vi "test_libssh2_session_callback_set.vi"() -> ()   [LabVIEW 2017, in "integration_tests.lvlib"]
uses:
  integration_tests.lvlib
  libssh2/libssh2_session_abstract.ctl
  libssh2/libssh2_session_callback_type.ctl
  libssh2/libssh2_session_handshake_tcp.vi
  libssh2/libssh2_init_default.vi
  <vilib>/Utility/tcp.llb/TCP Get Raw Net Object.vi
  libssh2/libssh2_session_handshake_socket.vi
  libssh2/libssh2_session_disconnect_ex.vi
  libssh2/libssh2.lvlib
  support/support.lvlib
  <vilib>/PNR/Transparent Assertions/Transparent Assertions/Transparent Assertions.lvlib
panel:
  out "error out":errorcluster
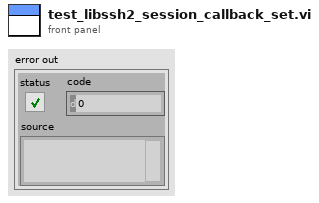
[diagram p1: front panel]
types:
  T1 = typedef "libssh2.lvlib/libssh2_session_abstract.ctl" = cluster{"send":refnum<vi>, "receive":refnum<vi>, "keyboard-interactive response":refnum<vi>}
  T2 = typedef "libssh2.lvlib/Session Refnum.ctl" = refnum<k1>
  T3 = typedef "libssh2.lvlib/libssh2_session_callback_type.ctl" = enum16{"Ignore", "Debug", "Disconnect", "MAC Error", "X11", "Send", "Receive", "Auth Agent", "Auth Agent Identities", "Auth Agent Sign"}
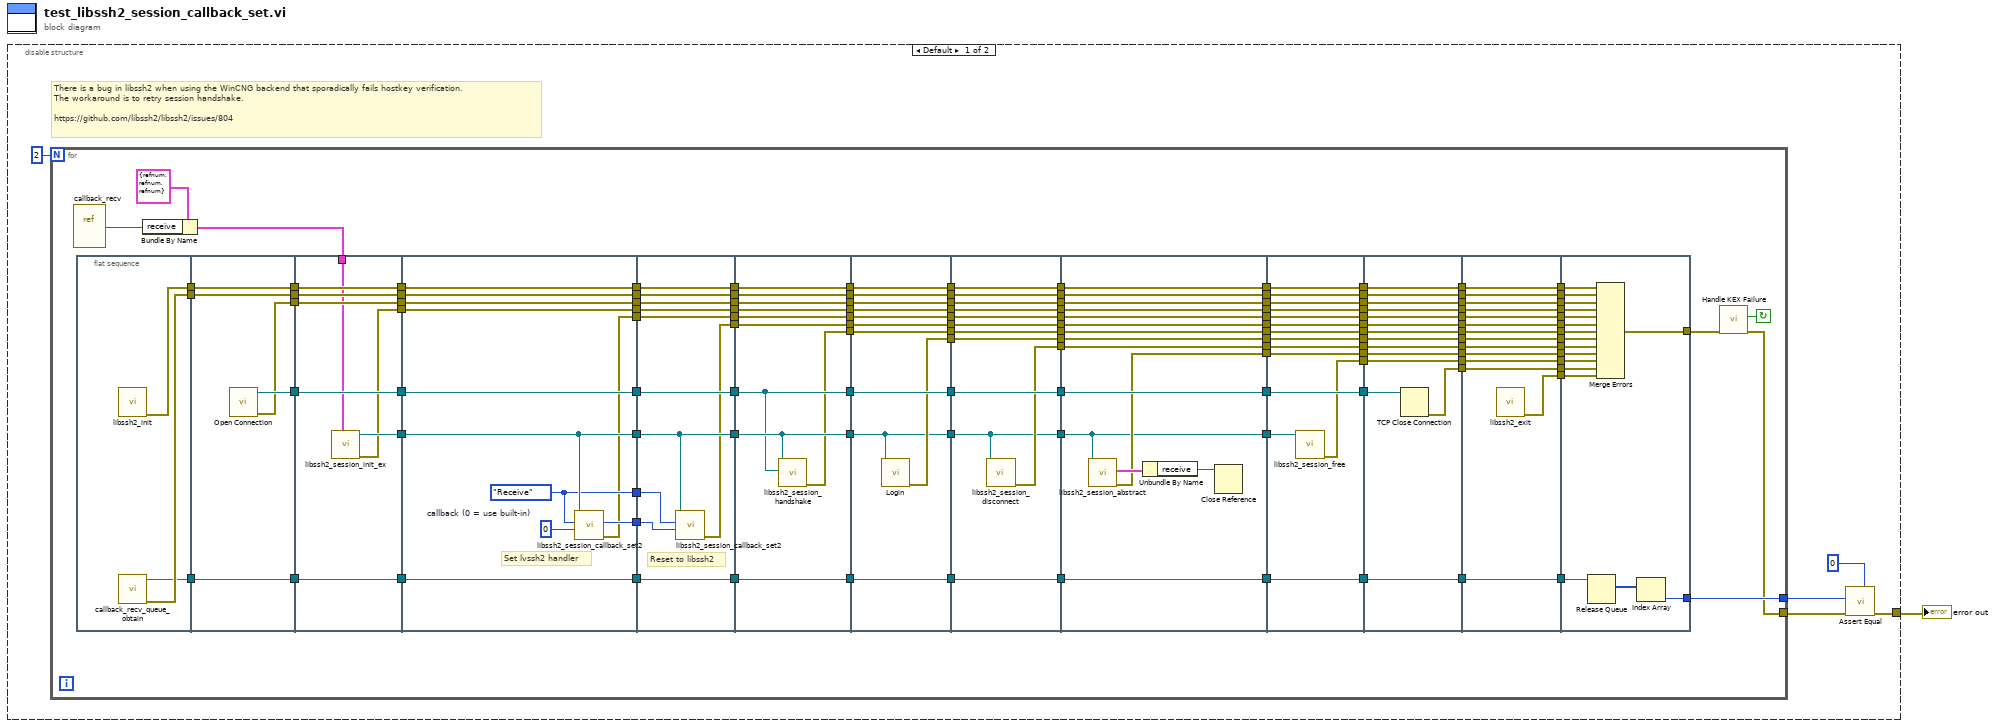
[diagram p0: block diagram]
diagram:
  n1 = disable-structure shown="Default" {
    disable-tunnel: [w5 _] -> w1
    frame condition #0 (active) {
      # "There is a bug in libssh2 when using the WinCNG backend that sporadically fails hostkey verification.\nThe workaround is to retry session handshake.\n\nhttps://github.com/libssh2/libssh2/issues/804"
      n2 = for {
        N: 2 -> [_]
        tunnel: [w10] -> w4
        tunnel: [w8] -> w3
        stop <- w7 continue-if-true
        n3 = vi-ref "callback_recv.vi"() -> (w12:refnum<vi>)
        n4 = flat-sequence {
          tunnel: [w136] -> w133
          tunnel: [w135] -> w132
          tunnel: [w134] -> w131
          tunnel: [w141] -> w130
          tunnel: w133 -> [w140]
          tunnel: [w140] -> w129
          tunnel: [w139] -> w128
          tunnel: w132 -> [w138]
          tunnel: [w138] -> w127
          tunnel: [w137] -> w126
          tunnel: w131 -> [w137]
          tunnel: w130 -> [w149]
          tunnel: [w149] -> w125
          tunnel: w129 -> [w148]
          tunnel: [w148] -> w124
          tunnel: w128 -> [w147]
          tunnel: [w147] -> w123
          tunnel: [w146] -> w122
          tunnel: [w145] -> w121
          tunnel: w127 -> [w144]
          tunnel: [w144] -> w120
          tunnel: w11 -> [w143]
          tunnel: [w142] -> w119
          tunnel: w126 -> [w142]
          tunnel: w125 -> [w160]
          tunnel: [w160] -> w118
          tunnel: w124 -> [w159]
          tunnel: [w159] -> w117
          tunnel: w123 -> [w158]
          tunnel: [w158] -> w116
          tunnel: w122 -> [w155]
          tunnel: [w155] -> w115
          tunnel: w121 -> [w157]
          tunnel: [w157] -> w114
          tunnel: w120 -> [w156]
          tunnel: [w156] -> w113
          tunnel: w119 -> [w154]
          tunnel: [w154] -> w112
          tunnel: [w153] -> w111
          tunnel: [w152] -> w110
          tunnel: [w151] -> w109
          tunnel: w118 -> [w171]
          tunnel: [w171] -> w108
          tunnel: w117 -> [w170]
          tunnel: [w170] -> w107
          tunnel: w116 -> [w169]
          tunnel: [w169] -> w106
          tunnel: w115 -> [w163]
          tunnel: [w163] -> w105
          tunnel: w114 -> [w168]
          tunnel: [w168] -> w104
          tunnel: w113 -> [w167]
          tunnel: [w167] -> w103
          tunnel: w112 -> [w166]
          tunnel: [w166] -> w102
          tunnel: w111 -> [w165]
          tunnel: w110 -> [w164]
          tunnel: w109 -> [w162]
          tunnel: [w162] -> w101
          tunnel: [w161] -> w100
          tunnel: w108 -> [w177]
          tunnel: [w177] -> w99
          tunnel: w107 -> [w181]
          tunnel: [w181] -> w98
          tunnel: w106 -> [w180]
          tunnel: [w180] -> w97
          tunnel: [w179] -> w96
          tunnel: w105 -> [w179]
          tunnel: w104 -> [w178]
          tunnel: [w178] -> w95
          tunnel: [w176] -> w94
          tunnel: w103 -> [w175]
          tunnel: [w175] -> w93
          tunnel: [w174] -> w92
          tunnel: w102 -> [w174]
          tunnel: w101 -> [w173]
          tunnel: [w173] -> w91
          tunnel: w100 -> [w172]
          tunnel: [w172] -> w90
          tunnel: w99 -> [w192]
          tunnel: [w192] -> w89
          tunnel: w98 -> [w191]
          tunnel: [w191] -> w88
          tunnel: w97 -> [w190]
          tunnel: [w190] -> w87
          tunnel: w96 -> [w185]
          tunnel: w95 -> [w189]
          tunnel: [w189] -> w86
          tunnel: w94 -> [w188]
          tunnel: [w188] -> w85
          tunnel: w93 -> [w187]
          tunnel: [w187] -> w84
          tunnel: [w186] -> w83
          tunnel: [w185] -> w82
          tunnel: [w184] -> w81
          tunnel: w92 -> [w184]
          tunnel: w91 -> [w183]
          tunnel: [w183] -> w80
          tunnel: w90 -> [w182]
          tunnel: [w182] -> w79
          tunnel: w89 -> [w204]
          tunnel: [w204] -> w78
          tunnel: w88 -> [w203]
          tunnel: [w203] -> w77
          tunnel: w87 -> [w202]
          tunnel: [w202] -> w76
          tunnel: w86 -> [w201]
          tunnel: [w201] -> w75
          tunnel: [w200] -> w74
          tunnel: w85 -> [w199]
          tunnel: [w199] -> w73
          tunnel: w84 -> [w198]
          tunnel: [w198] -> w72
          tunnel: w83 -> [w197]
          tunnel: [w197] -> w71
          tunnel: [w196] -> w70
          tunnel: w82 -> [w196]
          tunnel: [w195] -> w69
          tunnel: w81 -> [w195]
          tunnel: w80 -> [w194]
          tunnel: [w194] -> w68
          tunnel: w79 -> [w193]
          tunnel: [w193] -> w67
          tunnel: w78 -> [w219]
          tunnel: [w219] -> w66
          tunnel: w77 -> [w218]
          tunnel: [w218] -> w65
          tunnel: w76 -> [w217]
          tunnel: [w217] -> w64
          tunnel: w75 -> [w216]
          tunnel: [w216] -> w63
          tunnel: w74 -> [w215]
          tunnel: [w215] -> w62
          tunnel: w73 -> [w214]
          tunnel: [w214] -> w61
          tunnel: w72 -> [w213]
          tunnel: [w213] -> w60
          tunnel: w71 -> [w212]
          tunnel: [w212] -> w59
          tunnel: w70 -> [w208]
          tunnel: [w209] -> w58
          tunnel: [w208] -> w57
          tunnel: [w207] -> w56
          tunnel: w69 -> [w207]
          tunnel: w68 -> [w206]
          tunnel: [w206] -> w55
          tunnel: w67 -> [w205]
          tunnel: [w205] -> w54
          tunnel: w66 -> [w233]
          tunnel: [w233] -> w53
          tunnel: w65 -> [w232]
          tunnel: [w232] -> w52
          tunnel: w64 -> [w231]
          tunnel: [w231] -> w51
          tunnel: w63 -> [w230]
          tunnel: [w230] -> w50
          tunnel: w62 -> [w229]
          tunnel: [w229] -> w49
          tunnel: w61 -> [w228]
          tunnel: [w228] -> w48
          tunnel: w60 -> [w227]
          tunnel: [w227] -> w47
          tunnel: w59 -> [w226]
          tunnel: [w226] -> w46
          tunnel: w58 -> [w225]
          tunnel: [w225] -> w45
          tunnel: w57 -> [w224]
          tunnel: [w223] -> w44
          tunnel: [w222] -> w43
          tunnel: w56 -> [w222]
          tunnel: w55 -> [w221]
          tunnel: [w221] -> w42
          tunnel: w54 -> [w220]
          tunnel: [w220] -> w41
          tunnel: w53 -> [w247]
          tunnel: w52 -> [w246]
          tunnel: [w246] -> w40
          tunnel: w51 -> [w245]
          tunnel: [w245] -> w39
          tunnel: [w244] -> w38
          tunnel: w50 -> [w243]
          tunnel: [w243] -> w37
          tunnel: w49 -> [w242]
          tunnel: [w242] -> w36
          tunnel: w48 -> [w241]
          tunnel: [w241] -> w35
          tunnel: w47 -> [w240]
          tunnel: [w240] -> w34
          tunnel: w46 -> [w239]
          tunnel: [w239] -> w33
          tunnel: w45 -> [w238]
          tunnel: [w238] -> w32
          tunnel: [w237] -> w31
          tunnel: w44 -> [w237]
          tunnel: [w236] -> w30
          tunnel: w43 -> [w236]
          tunnel: w42 -> [w235]
          tunnel: [w235] -> w29
          tunnel: w41 -> [w234]
          tunnel: [w234] -> w28
          tunnel: w40 -> [w261]
          tunnel: [w261] -> w27
          tunnel: w39 -> [w260]
          tunnel: [w260] -> w26
          tunnel: w38 -> [w259]
          tunnel: [w259] -> w25
          tunnel: [w258] -> w24
          tunnel: w37 -> [w257]
          tunnel: [w257] -> w23
          tunnel: w36 -> [w256]
          tunnel: [w256] -> w22
          tunnel: w35 -> [w255]
          tunnel: [w255] -> w21
          tunnel: w34 -> [w254]
          tunnel: [w254] -> w20
          tunnel: w33 -> [w253]
          tunnel: [w253] -> w19
          tunnel: w32 -> [w252]
          tunnel: [w252] -> w18
          tunnel: [w251] -> w17
          tunnel: w31 -> [w251]
          tunnel: [w250] -> w16
          tunnel: w30 -> [w250]
          tunnel: w29 -> [w249]
          tunnel: [w249] -> w15
          tunnel: w28 -> [w248]
          tunnel: [w248] -> w14
          tunnel: w27 -> [w278]
          tunnel: w26 -> [w277]
          tunnel: w25 -> [w276]
          tunnel: w24 -> [w275]
          tunnel: w23 -> [w274]
          tunnel: w22 -> [w273]
          tunnel: w21 -> [w272]
          tunnel: w20 -> [w271]
          tunnel: w19 -> [w270]
          tunnel: w18 -> [w269]
          tunnel: w17 -> [w268]
          tunnel: w16 -> [w267]
          tunnel: w15 -> [w266]
          tunnel: w14 -> [w265]
          tunnel: [w263] -> w10
          tunnel: [w262] -> w9
          frame #0 {
            n5 = call-poly "libssh2_init.vi"() -> ("error out"=w136:errorcluster)  [unwired: 11 in]
            n6 = call "callback_recv_queue_obtain.vi"() -> ("error out"=w135:errorcluster, "queue out"=w134:refnum<queue>)  [unwired: 10 in]
          }
          frame #1 {
            n7 = call "Open Connection.vi"() -> ("error out"=w139:errorcluster, "connection ID"=w141:refnum<k5>)  [unwired: 10 in]
          }
          frame #2 {
            n8 = call "libssh2_session_init_ex.vi"("abstract"=w143) -> ("error out"=w145:errorcluster, "session"=w146:T2)  [unwired: 9 in]
          }
          frame #3 {
            w150 = u64 0  # callback (0 = use built-in)
            w153 = libssh2_session_callback_type."Receive" ("callback type")
            # "Set lvssh2 handler"
            n9 = call "libssh2_session_callback_set2.vi"("callback (0 = use built-in)"=w150, "callback type"=w153, "session"=w155) -> ("error out"=w151:errorcluster, "previous callback"=w152:u64)  [unwired: 7 in]
          }
          frame #4 {
            # "Reset to libssh2"
            n10 = call "libssh2_session_callback_set2.vi"("callback (0 = use built-in)"=w164, "callback type"=w165, "session"=w163) -> ("error out"=w161:errorcluster)  [unwired: 7 in, 1 out]
          }
          frame #5 {
            n11 = call-poly "libssh2_session_handshake.vi"("tcp connection"=w177, "session"=w179) -> ("error out"=w176:errorcluster)  [unwired: 9 in]
          }
          frame #6 {
            n12 = call "Login.vi"("session"=w185) -> ("error out"=w186:errorcluster)  [unwired: 10 in]
          }
          frame #7 {
            n13 = call "libssh2_session_disconnect.vi"("session"=w196) -> ("error out"=w200:errorcluster)  [unwired: 10 in]
          }
          frame #8 {
            n14 = call "libssh2_session_abstract.vi"("session"=w208) -> ("error out"=w209:errorcluster, "abstract"=w211:T1)  [unwired: 9 in]
            n15 = Unbundle By Name(w211) -> ("receive"=w210:refnum<vi>)
            n16 = Close Reference(reference=w210) -> ()  [unwired: 1 in, 1 out]
          }
          frame #9 {
            n17 = call "libssh2_session_free.vi"("session"=w224) -> ("error out"=w223:errorcluster)  [unwired: 10 in]
          }
          frame #10 {
            n18 = TCP Close Connection(connection ID=w247) -> (error out=w244:errorcluster)  [unwired: 2 in, 1 out]
          }
          frame #11 {
            n19 = call "libssh2_exit.vi"() -> ("error out"=w258:errorcluster)  [unwired: 11 in]
          }
          frame #12 {
            n20 = Release Queue(queue=w267) -> (remaining elements=w264:i32[])  [unwired: 2 in, 2 out]
            n21 = Merge Errors(w278, w271, w277, w274, w266, w265, w272, w270, w273, w269, w268, w276, w275) -> (w262:errorcluster)
            n22 = Index Array(array=w264) -> (element=w263:i32)  [unwired: 1 in]
          }
        }
        n23 = Bundle By Name(cluster=T1 {"send"=refnum, "receive"=refnum, "keyboard-interactive response"=refnum} ("abstract"), "receive"=w12) -> (w11:T1)
        n24 = call "Handle KEX Failure.vi"("error in (no error)"=w9) -> ("error out"=w8:errorcluster, "KEX Failure"=w7:bool)  [unwired: 9 in]
      }
      n25 = call <vilib>:"Assert Equal.vi"("Expected"=0 ("element"), "error in (no error)"=w3, "Actual"=w4) -> ("error out"=w5:errorcluster)  [unwired: 8 in]
    }
    frame condition #1 {
    }
  }
  "error out" <- w1
